vi "Clear-sequences.vi"(8 "error in (no error)":errorcluster, 11 "Available motors in":refnum<class "Motor-assembly.lvclass">) -> (0 "error out":errorcluster, 3 "Available motors out":refnum<class "Motor-assembly.lvclass">)   [LabVIEW 2013, in "PowderDeposition.lvlib" / "Motor-assembly.lvclass"]
uses:
  Motor-assembly.lvclass
  Motor-assembly.lvclass/Motor-assembly.ctl
  Sequence/Action-sequence.lvclass
  Motor/Motor.lvclass
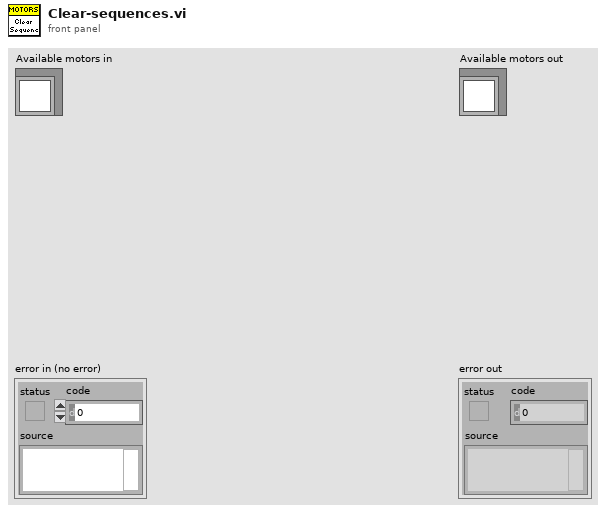
[diagram p1: front panel]
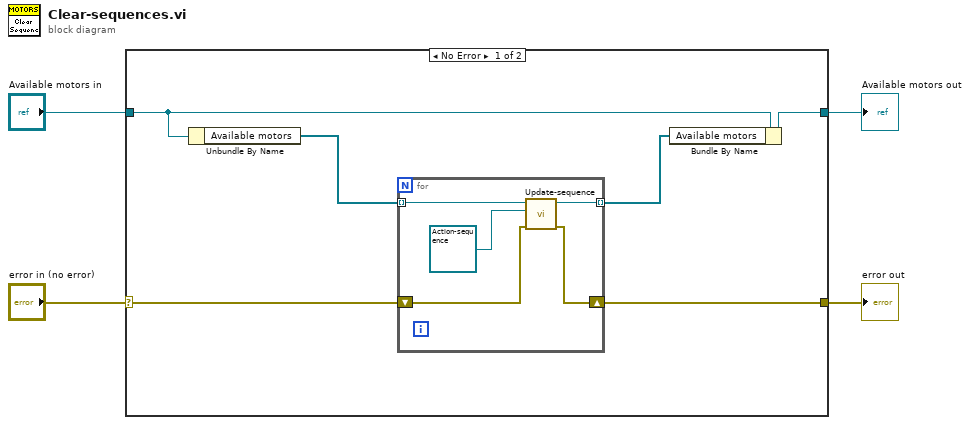
[diagram p0: block diagram]
diagram:
  n1 = case shown="No Error" "error in (no error)" {
    selector: "error in (no error)" -> [w5 w17]
    tunnel: [w6 w17] -> w3
    tunnel: [w9 w16] -> w1
    tunnel: "Available motors in" -> [w10 w16]
    frame No Error {
      n2 = Unbundle By Name(w10) -> ("Available motors"=w7:refnum<class "Motor.lvclass">[])
      n3 = for {
        tunnel: w7 -> [w15] mode=indexing
        tunnel: [w14] -> w8 mode=indexing
        shift-right: [w12] -> w6
        shift-left: w5 -> [w13]
        n4 = call-dynamic "Update-sequence.vi"("error in (no error)"=w13, "Sequence"=refnum<class "Action-sequence.lvclass"> refnum, "Motor in"=w15) -> ("error out"=w12:errorcluster, "Motor out"=w14:refnum<class "Motor.lvclass">)  [unwired: 7 in]
      }
      n5 = Bundle By Name(cluster=w10, "Available motors"=w8) -> (w9:refnum<class "Motor-assembly.lvclass">)
    }
    frame Error {
    }
  }
  "error out" <- w3
  "Available motors out" <- w1
